vi "Create Connection.vi"(8 "error in (no error)":errorcluster caption="错误输入（无错误）", 11 "connectionString":string) -> (0 "error out":errorcluster caption="错误输出", 3 "OleDBClass 输出":refnum<class "OleDBClass.lvclass"> caption="DNL_LabVIEW Object out")   [LabVIEW 2012, in "OleDBClass.lvclass"]
uses:
  OleDBClass.lvclass
  System.Data
  OleDBClass.lvclass/OleDBClass.ctl
panel:
  in  "OleDBClass 输入":refnum<class "OleDBClass.lvclass"> caption="DNL_LabVIEW Object in"
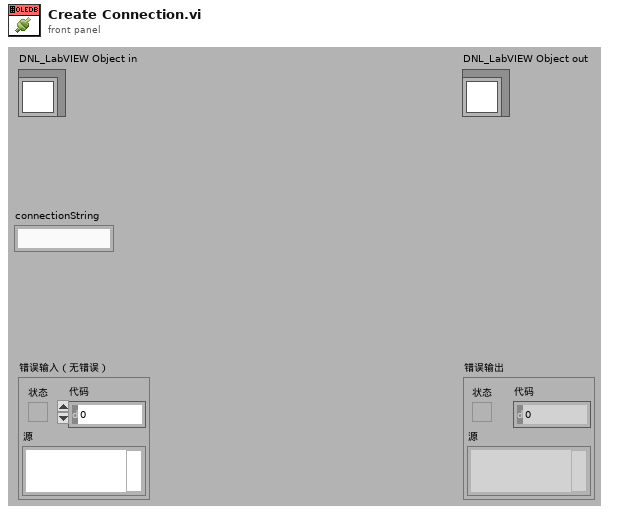
[diagram p1: front panel]
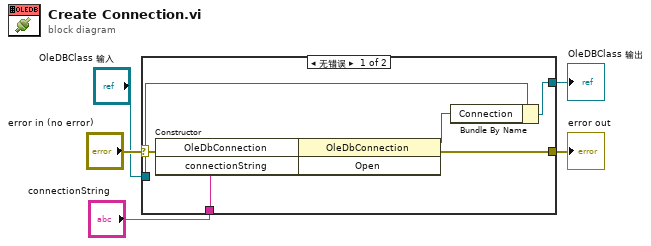
[diagram p0: block diagram]
diagram:
  n1 = case shown="无错误" "error in (no error)" {
    selector: "error in (no error)" -> [w11 w15]
    tunnel: [w6 w15] -> w4
    tunnel: [w12 w14] -> w2
    tunnel: "OleDBClass 输入" -> [w13 w14]
    tunnel: "connectionString" -> [w10 _]
    frame No Error {
      n2 = constructor class="OleDbConnection"(error in=w11, "connectionString"=w10) -> (reference out=w8:refnum<k24>, error out=w9:errorcluster)  [unwired: 2 in, 2 out]
      n3 = invoke class="OleDbConnection" method="Open"(reference=w8, error in=w9) -> (reference out=w7:refnum<k24>, error out=w6:errorcluster)  [unwired: 1 in, 1 out]
      n4 = Bundle By Name(cluster=w13, "Connection"=w7) -> (w12:refnum<class "OleDBClass.lvclass">)
    }
    frame Error {
    }
  }
  "error out" <- w4
  "OleDBClass 输出" <- w2
